vi "startedGlobal.vi"(9 "started":bool=TRUE, 10 "Action":enum16{"Write", "Read", "Reset"}(ring)) -> (1 "started?":bool)   [LabVIEW 2009, in "Hardware.lvlib" / "Channels.lvlib" / "DIO64Output.lvclass"]
uses:
  DIO64Output.lvclass
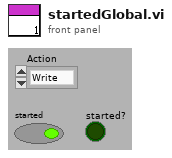
[diagram p1: front panel]
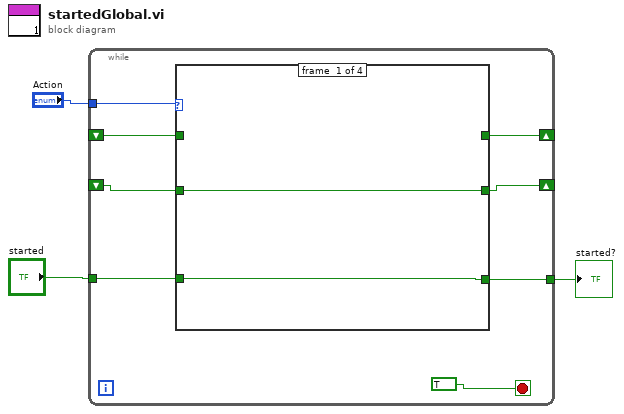
[diagram p0: block diagram]
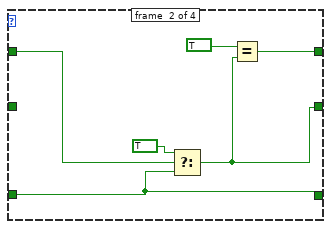
[diagram p2: hidden frame]
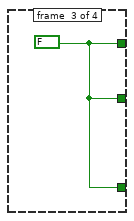
[diagram p3: hidden frame]
diagram:
  n1 = while {
    tunnel: "Action" -> [w11]
    shift-right: [w6] -> _
    shift-left: _ -> [w8]
    tunnel: "started" -> [w9]
    tunnel: [w7] -> w1
    shift-right: [w5] -> _
    shift-left: _ -> [w4]
    stop <- TRUE stop-if-true
    n2 = case shown="\"Reset\"" w11 {
      tunnel: [w13 w16 w20 w22] -> w6
      tunnel: w9 -> [w12 w15 _ _]
      tunnel: w8 -> [w13 _ _ w22]
      tunnel: [w12 w15 w20 w22] -> w7
      tunnel: [_ w18 w20 w21] -> w5
      tunnel: w4 -> [_ w17 _ w21]
      frame #0 {
      }
      frame #1 {
        n3 = Select(t=TRUE, s=w17, f=w15) -> (s? t:f=w16:bool)
        n4 = Equal?(x=TRUE, y=w16) -> (x = y?=w18:bool)
      }
      frame #2 {
        w20 = FALSE
      }
      frame #3 {
      }
    }
  }
  "started?" <- w1
